vi "DEV test VIs unwrapped.vi"() -> ()   [LabVIEW 2018, in "Image Management.lvlib"]
uses:
  Action.ctl
  Image Management.lvlib
panel:
  out "Rows Where Whitespace Starts":i32[](array[numeric])
  out "Image Pixels (I16)":i16[][](array[numeric])
  out "Error Out":errorcluster
  in  "Error In":errorcluster
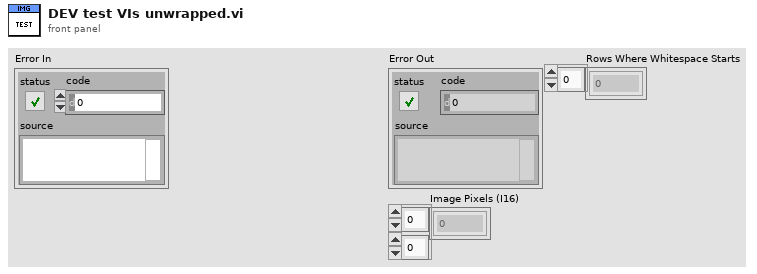
[diagram p1: front panel]
types:
  T1 = typedef "Image Management.lvlib/Action.ctl" = enum16{"Init", "Find Linespaces", "Close"}
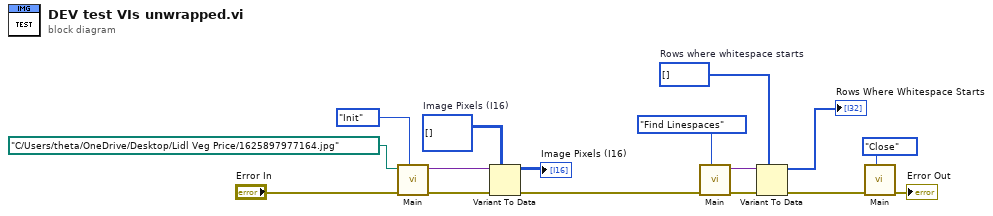
[diagram p0: block diagram]
diagram:
  w7 = i16[][] []  # Image Pixels (I16)
  w9 = i32[] []  # Rows where whitespace starts
  n1 = call "Main.vi"("Action"=Action."Init", "Error In"="Error In", "File Path to Load"=path "C:/Users/theta/OneDrive/Desktop/Lidl Veg Price/1625897977164.jpg" ("File Path")) -> ("Error Out"=w4:errorcluster, "Output"=w8:variant)  [unwired: 7 in]
  n2 = Variant To Data(error in=w4, type=w7, Variant=w8) -> (data=→"Image Pixels (I16)":i16[][], error out=w3:errorcluster)
  n3 = call "Main.vi"("Action"=Action."Find Linespaces", "Error In"=w3) -> ("Error Out"=w2:errorcluster, "Output"=w10:variant)  [unwired: 8 in]
  n4 = Variant To Data(error in=w2, type=w9, Variant=w10) -> (data=→"Rows Where Whitespace Starts":i32[], error out=w1:errorcluster)
  n5 = call "Main.vi"("Action"=Action."Close", "Error In"=w1) -> ("Error Out"=→"Error Out":errorcluster)  [unwired: 8 in, 1 out]
